vi "Write average.vi"(10 "average":i32, 11 "ValveModbus in":refnum<class "NeedleValve.lvclass">) -> (3 "ValveModbus out":refnum<class "NeedleValve.lvclass">)   [LabVIEW 2019, in "NeedleValve.lvclass"]
uses:
  NeedleValve.lvclass
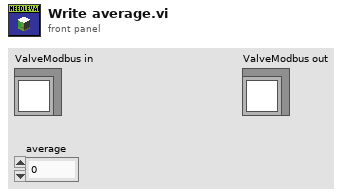
[diagram p1: front panel]
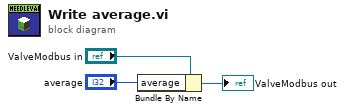
[diagram p0: block diagram]
diagram:
  n1 = Bundle By Name(cluster="ValveModbus in", "average"="average") -> (→"ValveModbus out":refnum<class "NeedleValve.lvclass">)
